vi "ValidacaoPontos.vi"(10 "TempoEntrePontos":dbl, 11 "Pontos":dbl[](array[numeric])) -> (0 "error out":errorcluster)   [LabVIEW 2019]
uses:
  TelaConfig/Configuracao.Variaveis.vi
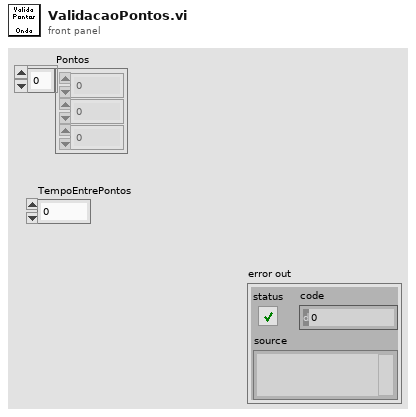
[diagram p1: front panel]
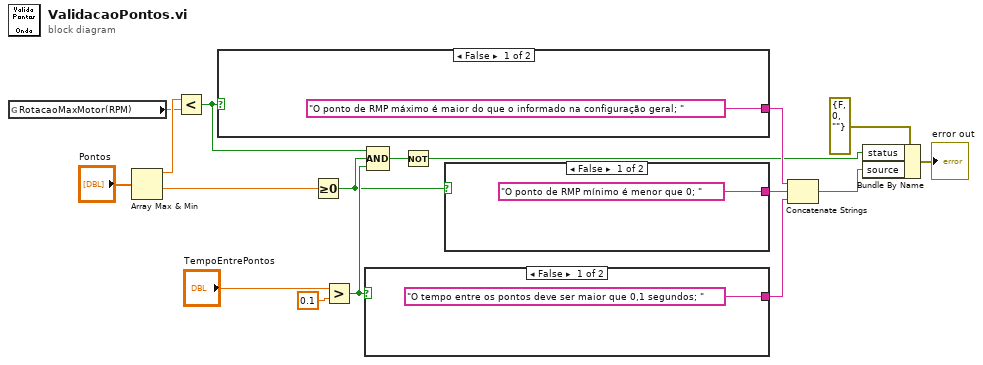
[diagram p0: block diagram]
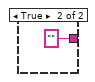
[diagram p2: hidden frame]
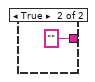
[diagram p3: hidden frame]
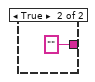
[diagram p4: hidden frame]
diagram:
  n1 = global read "Configuracao.Variaveis.vi" "RotacaoMaxMotor(RPM)"() -> (w12:dbl)
  n2 = Array Max & Min(array="Pontos") -> (max value=w13:dbl, min value=w14:dbl)  [unwired: 2 out]
  n3 = Less?(x=w13, y=w12) -> (x < y?=w11:bool)
  n4 = case shown="False" w11 {
    tunnel: ["O ponto de RMP máximo é maior do que o informado na configuração geral; " ""] -> w8
    frame False {
    }
    frame True {
    }
  }
  n5 = Greater Or Equal To 0?(x=w14) -> (x >= 0?=w9:bool)
  n6 = Greater?(x="TempoEntrePontos", y=0.1) -> (0:w10:bool)
  n7 = case shown="False" w10 {
    tunnel: ["O tempo entre os pontos deve ser maior que 0,1 segundos; " ""] -> w6
    frame False {
    }
    frame True {
    }
  }
  n8 = Compound Arithmetic op=AND(w11, w9, w10) -> (w3:bool)
  n9 = Not(x=w3) -> (.not. x?=w1:bool)
  n10 = case shown="False" w9 {
    tunnel: ["O ponto de RMP mínimo é menor que 0; " ""] -> w7
    frame False {
    }
    frame True {
    }
  }
  n11 = Concatenate Strings(w8, w7, w6) -> (w2:string)
  n12 = Bundle By Name(cluster=errorcluster {"status"=FALSE, "code"=0, "source"=""} ("error out"), "status"=w1, "source"=w2) -> (→"error out":errorcluster)
